vi "LEBITplc.FileTo2dArray.vi"(2 "file path (dialog if empty)":path, 4 "Create if ness.":bool, 5 "error in":errorcluster) -> (17 "Array":string[][](array[string]), 19 "error out":errorcluster)   [LabVIEW 2014, in "LEBITplc.lvlib"]
uses:
  LEBITplc.lvlib
  CS_Core/CSSystem/CoreDefs/CoreDefs.error_type.ctl
  CS_Core/CSSystem/CoreDefs/CoreDefs.error_severity.ctl
  CS_Core/CSSystem/CoreLib/CoreLib.lvlib
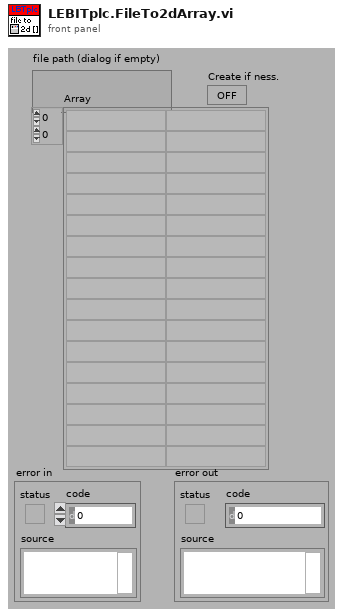
[diagram p1: front panel]
types:
  T1 = typedef "CoreDefs.error_severity.ctl" = enum16{"undefined", "information", "warning", "error", "fatal"}
  T2 = typedef "CoreDefs.error_type.ctl" = enum16{"no error", "can't load process", "can't unload process", "process does not exist", "can't install process", "can't remove process", "unknown function", "time out", "can't execute function", "duplicate queue name", "super not found", "caller queue invalid", "can't ping process", "unknown error", "VISA Error", "VISA timeout", "GPIB timeout", "GPIB error", "communication error", "data type mismatch", "can't read data from OPC server", "can't write data to OPC server", "OET error", "function not implemented", "process already exists", "invalid Shared Variable name", "error writing Shared Variable", "error reading Shared Variable", "invalid client name", "corrupt database", "unknown class", "call not authorized", "parameter out of range", "OET timeout: can't get data to modify", "invalid queue name", "requested operation incompatible with current state", "event undefined", "event disabled", "state undefined", "caller is not a friend", "EventBuilder: bad eventID", "EventBuilder: no DAQ devices", "a thread must not stop itself", "UNUSED ELEMENT4", "DiscArchiver: eventData incomplete", "DiscArchiver: eventData does not belong to run", "DiscArchiver: can't open file", "DiscArchiver: can't write to file", "DiscArchiver: available disc space low", "can't acquire semaphore", "error reading data from database", "notifier object is not existing", "can't register process", "can't unregister process", "illegal event type", "object disabled", "object already exists", "can't change state", "Instrument not found", "no connection to remote node", "invalid reference", "N/A", "UNUSED ELEMENT 1", "element not found", "illegal TCP/IP connection detected", "object does not exist", "invalid access ID", "unknown CS system", "invalid privilige", "unsupported data type", "unsupported server type", "IO server already exists", "Shared Variable already exists"}
  T3 = enum16{"open", "replace", "create", "open or create", "replace or create", "replace or create with confirmation"}
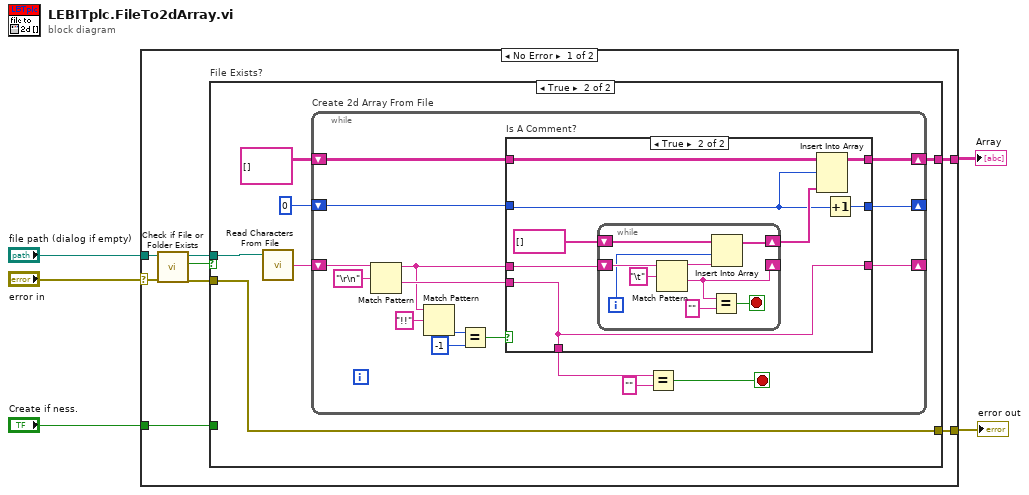
[diagram p0: block diagram]
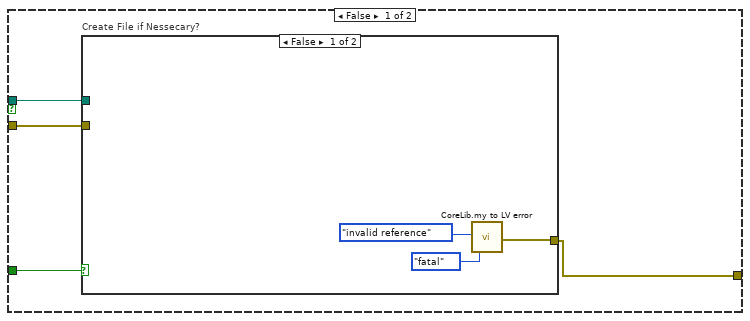
[diagram p2: hidden frame]
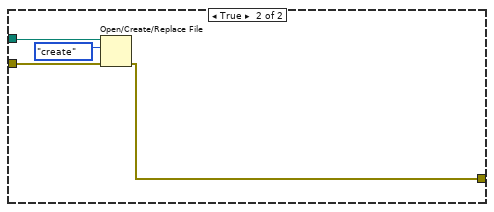
[diagram p3: hidden frame]
diagram:
  n1 = case shown="No Error" "error in" {
    selector: "error in" -> [w9 w67]
    tunnel: "file path (dialog if empty)" -> [w13 _]
    tunnel: [w8 _] -> w3
    tunnel: [w7 w67] -> w2
    tunnel: "Create if ness." -> [w6 _]
    frame No Error {
      n2 = call <vilib>:"Check if File or Folder Exists.vi"("error in (no error)"=w9, "path"=w13) -> ("error out"=w10:errorcluster, "file or folder exists?"=w11:bool, "dup path"=w12:path)  [unwired: 7 in]
      n3 = case "File Exists?" shown="True" w11 {
        tunnel: w12 -> [w17 w28]
        tunnel: [_ w27] -> w8
        tunnel: w10 -> [w16 w26]
        tunnel: [w15 w26] -> w7
        tunnel: w6 -> [w14 _]
        frame False {
          n4 = case "Create File if Nessecary?" shown="False" w14 {
            tunnel: w17 -> [_ w23]
            tunnel: w16 -> [_ w22]
            tunnel: [w18 w21] -> w15
            frame False {
              n5 = call "CoreLib.my to LV error.vi"("ErrorTypes"=CoreDefs.error_type."invalid reference", "severityLevel"=CoreDefs.error_severity."fatal") -> ("myErrorCluster"=w18:errorcluster)  [unwired: 16 in, 1 out]
            }
            frame True {
              n6 = Open/Create/Replace File(file path (use dialog)=w23, error in=w22, operation (0:open)=T3."create") -> (error out=w21:errorcluster)  [unwired: 3 in, 2 out]
            }
          }
        }
        frame True {
          n7 = call <vilib>:"Read Characters From File.vi"("file path (dialog if empty)"=w28) -> ("character string"=w30:string)  [unwired: 5 in, 3 out]
          n8 = while "Create 2d Array From File" {
            shift-right: [w36] -> _
            shift-left: w30 -> [w46]
            shift-right: [w44] -> w27
            shift-left: string[][] [] -> [w43]
            shift-right: [w34] -> _
            shift-left: 0 -> [w35]
            stop <- w32 stop-if-true
            n9 = Match Pattern(string=w46, regular expression="\r\n") -> (before substring=w41:string, after substring=w42:string)  [unwired: 1 in, 2 out]
            n10 = Match Pattern(string=w41, regular expression="!!") -> (offset past match=w39:i32)  [unwired: 1 in, 3 out]
            n11 = Equal?(x=w39, y=-1) -> (x = y?=w37:bool)
            n12 = case "Is A Comment?" shown="True" w37 {
              tunnel: [w48 w56] -> w44
              tunnel: w43 -> [w48 w55]
              tunnel: w42 -> [w47 w50]
              tunnel: w41 -> [_ w53]
              tunnel: [w47 w50] -> w36
              tunnel: w35 -> [w49 w52]
              tunnel: [w49 w51] -> w34
              tunnel: [w47 w50] -> w31
              frame False {
              }
              frame True {
                n13 = while {
                  shift-right: [w60] -> _
                  shift-left: w53 -> [w66]
                  shift-right: [w61] -> w54
                  shift-left: string[] [] -> [w64]
                  i -> [w62]
                  stop <- w58 stop-if-true
                  n14 = Match Pattern(string=w66, regular expression="\t") -> (before substring=w63:string, after substring=w60:string)  [unwired: 1 in, 2 out]
                  n15 = Equal?(x=w60, y="") -> (x = y?=w58:bool)
                  n16 = Insert Into Array(array=w64, index=w62, new element=w63) -> (w61:string[])
                }
                n17 = Insert Into Array(array=w55, index (row)=w52, new element=w54) -> (w56:string[][])  [unwired: 1 in]
                n18 = Increment(x=w52) -> (x+1=w51:i32)
              }
            }
            n19 = Equal?(x=w31, y="") -> (x = y?=w32:bool)
          }
        }
      }
    }
    frame Error {
    }
  }
  "Array" <- w3
  "error out" <- w2
